vi "INIT.vi"(7 "error in (no error)":errorcluster, 10 "Control-Client in":refnum<class "Control-Client.lvclass">) -> (0 "error out":errorcluster, 3 "Control-Client out":refnum<class "Control-Client.lvclass">)   [LabVIEW 2015]
uses:
  Classes/Control/Control-Client/Control-Client.lvclass
  Classes/Config/Config.lvclass
  Classes/Config/config_names_def.ctl
  Classes/GeneralFunctionality/GeneralFunctionality.lvclass/GeneralFunctionality.ctl
  Classes/Control/Control-Client/Control-Client.lvclass/Control-Client.ctl
  Clusters-def/Message types.ctl
  Classes/Message/Message.lvclass
  Classes/Message/Message.lvclass/Message.ctl
  Classes/GeneralFunctionality/GeneralFunctionality.lvclass
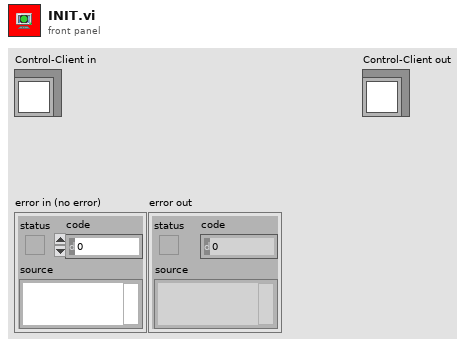
[diagram p1: front panel]
types:
  T1 = typedef "Config.lvclass/config_names_def.ctl" = string
  T2 = typedef "Message types.ctl" = string
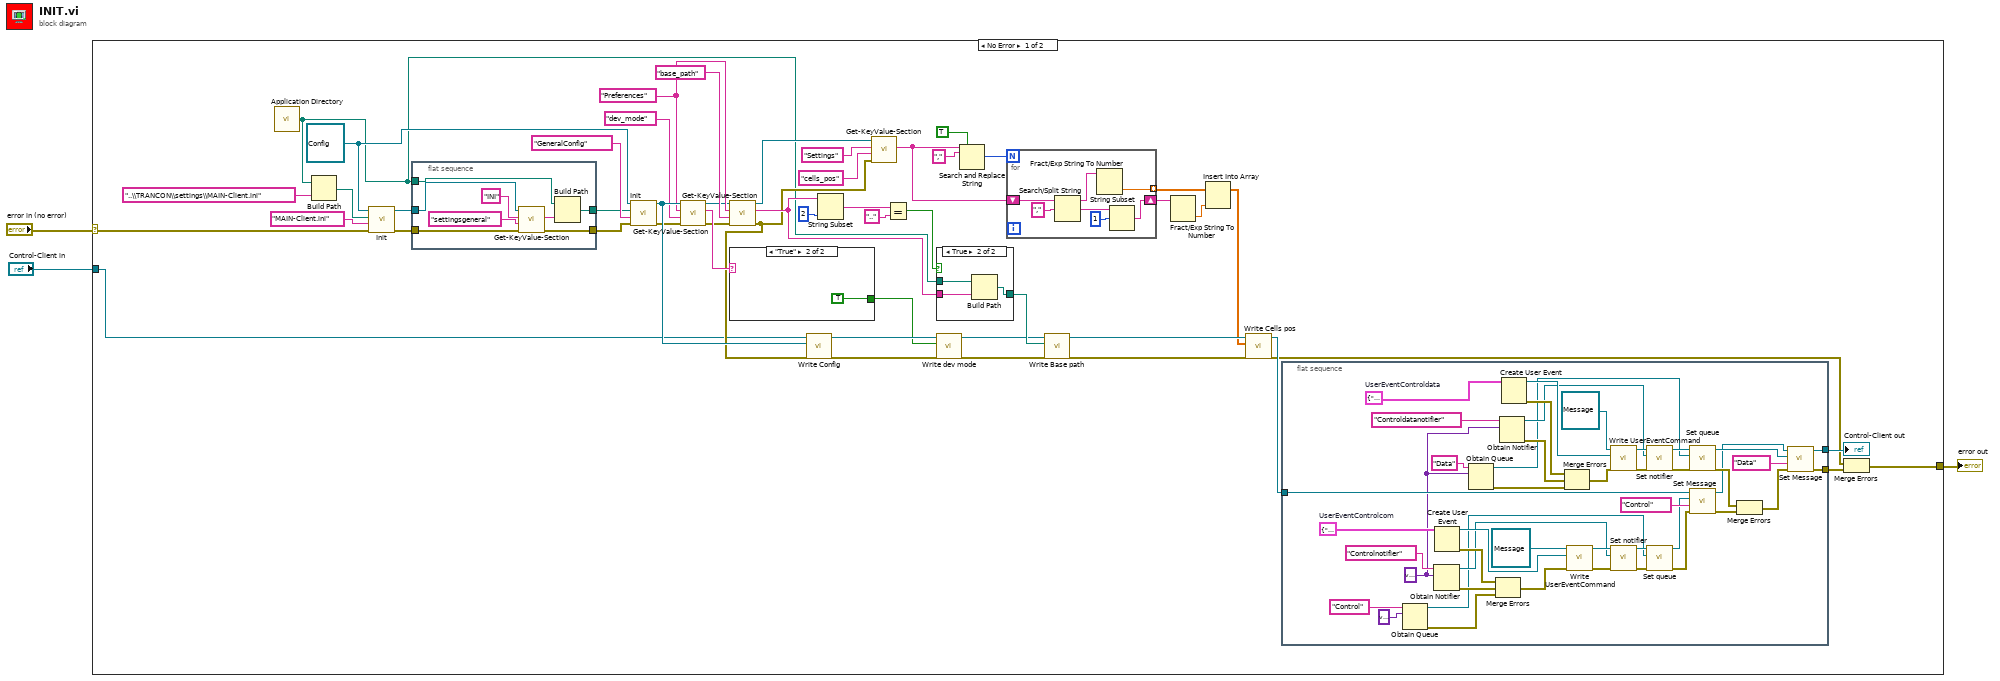
[diagram p0: block diagram]
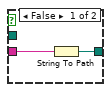
[diagram p2: hidden frame]
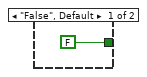
[diagram p3: hidden frame]
diagram:
  n1 = case shown="No Error" "error in (no error)" {
    selector: "error in (no error)" -> [w24 w120]
    tunnel: [w35 w120] -> w3
    tunnel: "Control-Client in" -> [w4 _]
    frame No Error {
      w34 = "Preferences" ("Section")
      w47 = refnum<class "Config.lvclass"> refnum ("Config.lvclass")
      n2 = call <vilib>:"Application Directory.vi"() -> ("Application Directory"=w5:path)
      n3 = Build Path(base path=w5, name or relative path="..\\TRANCON\\settings\\MAIN-Client.ini" ("nom ou chemin relatif")) -> (appended path=w51:path)
      n4 = call "Init.vi"("error in"=w24, "Name"="MAIN-Client.ini", "Path"=w51, "Config in"=w47) -> ("error out"=w49:errorcluster, "Config out"=w50:refnum<class "Config.lvclass">)  [unwired: 6 in]
      n5 = flat-sequence {
        tunnel: w50 -> [w119]
        tunnel: w49 -> [w118]
        tunnel: w5 -> [w114]
        tunnel: [w113] -> w45
        tunnel: [w112] -> w46
        frame #0 {
          n6 = call-dynamic "Get-KeyValue-Section.vi"("error in (no error)"=w118, "Key"="settingsgeneral", "Section"="INI", "Config in"=w119) -> ("error out"=w113:errorcluster, "Value"=w115:string)  [unwired: 5 in, 1 out]
          n7 = Build Path(base path=w114, name or relative path=w115) -> (appended path=w112:path)
        }
      }
      n8 = call "Init.vi"("error in"=w45, "Name"=T1 "GeneralConfig" ("Combo Box"), "Path"=w46, "Config in"=w47) -> ("error out"=w42:errorcluster, "Config out"=w44:refnum<class "Config.lvclass">)  [unwired: 6 in]
      n9 = call-dynamic "Get-KeyValue-Section.vi"("error in (no error)"=w42, "Key"="dev_mode", "Section"=w34, "Config in"=w44) -> ("error out"=w32:errorcluster, "Value"=w41:string, "Config out"=w31:refnum<class "Config.lvclass">)  [unwired: 5 in]
      n10 = call-dynamic "Get-KeyValue-Section.vi"("error in (no error)"=w32, "Key"="base_path", "Section"=w34, "Config in"=w31) -> ("error out"=w14:errorcluster, "Value"=w26:string, "Config out"=w17:refnum<class "Config.lvclass">)  [unwired: 5 in]
      n11 = case shown="\"True\"" w41 {
        tunnel: [FALSE TRUE] -> w38
        frame "False", Default {
        }
        frame "True" {
        }
      }
      n12 = call "Write Config.vi"("error in (no error)"=w14, "Config.lvclass"=w44, "GeneralFunctionality en entrée"=w4) -> ("error out"=w40:errorcluster, "GeneralFunctionality en sortie"=w39:refnum<class "Control-Client.lvclass">)  [unwired: 7 in]
      n13 = String Subset(string=w26, length (rest)=2 ("length (rest)")) -> (substring=w29:string)  [unwired: 1 in]
      n14 = call-dynamic "Get-KeyValue-Section.vi"("error in (no error)"=w14, "Key"="cells_pos", "Section"="Settings", "Config in"=w17) -> ("Value"=w7:string)  [unwired: 5 in, 2 out]
      n15 = Equal?(x=w29, y=".." ("x")) -> (x = y?=w27:bool)
      n16 = case shown="True" w27 {
        tunnel: w5 -> [_ w65]
        tunnel: w26 -> [w62 w64]
        tunnel: [w61 w63] -> w25
        frame False {
          n17 = String To Path(string=w62) -> (path=w61:path)
        }
        frame True {
          n18 = Build Path(base path=w65, name or relative path=w64) -> (appended path=w63:path)
        }
      }
      n19 = call "Write dev mode.vi"("error in (no error)"=w40, "Dev_mode"=w38, "Control-Client in"=w39) -> ("error out"=w22:errorcluster, "Control-Client out"=w23:refnum<class "Control-Client.lvclass">)  [unwired: 7 in]
      n20 = Search and Replace String(replace all?=TRUE ("replace all? (F)"), input string=w7, search string=",") -> (number of replacements=w12:i32)  [unwired: 5 in, 3 out]
      n21 = for {
        N: w12 -> [_]
        tunnel: [w54] -> w10 mode=indexing
        shift-right: [w56] -> w9
        shift-left: w7 -> [w59]
        n22 = Search/Split String(string=w59, search string/char (-)=",") -> (substring before match=w55:string, match + rest of string=w58:string)  [unwired: 1 in, 1 out]
        n23 = Fract/Exp String To Number(string=w55) -> (number=w54:dbl)  [unwired: 3 in, 1 out]
        n24 = String Subset(string=w58, offset (0)=1) -> (substring=w56:string)  [unwired: 1 in]
      }
      n25 = call "Write Base path.vi"("error in (no error)"=w22, "Base path"=w25, "Control-Client in"=w23) -> ("error out"=w21:errorcluster, "Control-Client out"=w20:refnum<class "Control-Client.lvclass">)  [unwired: 7 in]
      n26 = Fract/Exp String To Number(string=w9) -> (number=w8:dbl)  [unwired: 3 in, 1 out]
      n27 = Insert Into Array(array=w10, new element=w8) -> (w6:dbl[])  [unwired: 1 in]
      n28 = call "Write Cells pos.vi"("error in (no error)"=w21, "Cells pos"=w6, "Control-Client in"=w20) -> ("error out"=w18:errorcluster, "Control-Client out"=w19:refnum<class "Control-Client.lvclass">)  [unwired: 7 in]
      n29 = flat-sequence {
        tunnel: w19 -> [w70]
        tunnel: [w69] -> w37
        tunnel: [w68] -> w36
        frame #0 {
          w90 = cluster{"command":string, "data":variant} {"command"="", "data"=variant}  # UserEventControldata
          w66 = variant
          w105 = cluster{"command":string, "data":variant} {"command"="", "data"=variant}  # UserEventControlcom
          n30 = Obtain Queue(name (unnamed)="Control", element data type=variant) -> (queue out=w80:refnum<queue>, error out=w86:errorcluster)  [unwired: 3 in, 1 out]
          n31 = Obtain Notifier(name (unnamed)="Controlnotifier" ("nom (aucun)"), notification data type=w66) -> (notifier out=w101:refnum<notifier>, error out=w102:errorcluster)  [unwired: 2 in, 1 out]
          n32 = Create User Event(user event datatype=w105) -> (user event=w107:refnum<user-event>, error out=w103:errorcluster)  [unwired: 1 in]
          n33 = Obtain Queue(name (unnamed)="Data", element data type=w66) -> (queue out=w79:refnum<queue>, error out=w85:errorcluster)  [unwired: 3 in, 1 out]
          n34 = Merge Errors(w103, w102, w86) -> (w100:errorcluster)
          n35 = Obtain Notifier(name (unnamed)="Controldatanotifier" ("nom (aucun)"), notification data type=w66) -> (notifier out=w82:refnum<notifier>, error out=w87:errorcluster)  [unwired: 2 in, 1 out]
          n36 = Create User Event(user event datatype=w90) -> (user event=w83:refnum<user-event>, error out=w88:errorcluster)  [unwired: 1 in]
          n37 = Merge Errors(w88, w87, w85) -> (w84:errorcluster)
          n38 = call "Write UserEventCommand.vi"("error in (no error)"=w100, "UserEventCommand"=w107, "Message en entrée"=refnum<class "Message.lvclass"> refnum ("Message.lvclass")) -> ("error out"=w104:errorcluster, "Message en sortie"=w108:refnum<class "Message.lvclass">)  [unwired: 7 in]
          n39 = call "Write UserEventCommand.vi"("error in (no error)"=w84, "UserEventCommand"=w83, "Message en entrée"=refnum<class "Message.lvclass"> refnum ("Message.lvclass")) -> ("error out"=w94:errorcluster, "Message en sortie"=w93:refnum<class "Message.lvclass">)  [unwired: 7 in]
          n40 = call "Set notifier.vi"("error in (no error)"=w104, "notifier"=w101, "Message en entrée"=w108) -> ("error out"=w97:errorcluster, "Message en sortie"=w98:refnum<class "Message.lvclass">)  [unwired: 7 in]
          n41 = call "Set notifier.vi"("error in (no error)"=w94, "notifier"=w82, "Message en entrée"=w93) -> ("error out"=w81:errorcluster, "Message en sortie"=w91:refnum<class "Message.lvclass">)  [unwired: 7 in]
          n42 = call "Set queue.vi"("error in (no error)"=w97, "queue"=w80, "Message in"=w98) -> ("error out"=w75:errorcluster, "Message out"=w73:refnum<class "Message.lvclass">)  [unwired: 7 in]
          n43 = call "Set queue.vi"("error in (no error)"=w81, "queue"=w79, "Message in"=w91) -> ("error out"=w78:errorcluster, "Message out"=w72:refnum<class "Message.lvclass">)  [unwired: 7 in]
          n44 = call "Set Message.vi"("error in (no error)"=w75, "Message type"=T2 "Control", "Message.lvclass"=w73, "GeneralFunctionality en entrée"=w70) -> ("error out"=w76:errorcluster, "GeneralFunctionality en sortie"=w71:refnum<class "Control-Client.lvclass">)  [unwired: 6 in]
          n45 = Merge Errors(w78, w76) -> (w77:errorcluster)
          n46 = call "Set Message.vi"("error in (no error)"=w77, "Message type"=T2 "Data", "Message.lvclass"=w72, "GeneralFunctionality en entrée"=w71) -> ("error out"=w68:errorcluster, "GeneralFunctionality en sortie"=w69:refnum<class "Control-Client.lvclass">)  [unwired: 6 in]
        }
      }
      n47 = Merge Errors(w18, w36) -> (w35:errorcluster)
      "Control-Client out" <- w37
    }
    frame Error {
    }
  }
  "error out" <- w3
